vi "Main Application Instance VIs.vi"(8 "Error In":errorcluster, 11 "App In":refnum<vi>) -> (0 "Error Out":errorcluster, 2 "VIs":T1[](array[typedef]), 3 "App Out":refnum<vi>)   [LabVIEW 2017, in "Bookmark Manager.lvlib"]
doc: "According to LabVIEW help: \"LabVIEW also creates a main application instance [MAI], which contains open VIs that are not part of a project and VIs that you did not open from a project.\""
uses:
  Bookmark Manager.lvlib
  Controls/VI Information.ctl
  Controls/Application Information.ctl
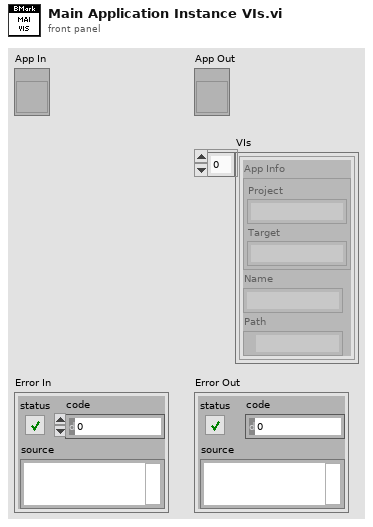
[diagram p1: front panel]
types:
  T1 = typedef "Bookmark Manager.lvlib/VI Information.ctl" = cluster{"App Info":T2, "Name":string, "Path":path}
  T2 = typedef "Bookmark Manager.lvlib/Application Information.ctl" = cluster{"Project":string, "Target":string}
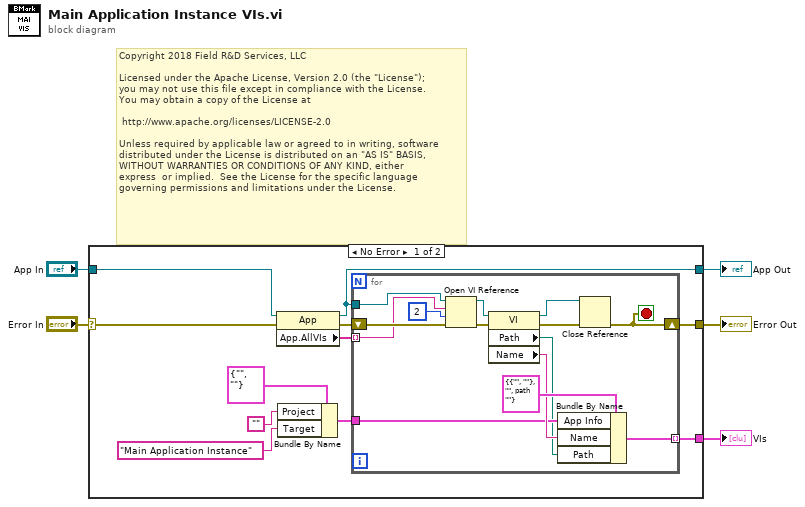
[diagram p0: block diagram]
diagram:
  # "Copyright 2018 Field R&D Services, LLC\n\nLicensed under the Apache License, Version 2.0 (the \"License\");\nyou may not use this file except in compliance with the License.\nYou may obtain a copy of the License at\n\n\thttp://www.apache.org/licenses/LICENSE-2.0\n\nUnless required by applicable law or agreed to in writing, software\ndistributed under the License is distributed on an \"AS IS\" BASIS,\nWITHOUT WARRANTIES OR CONDITIONS OF ANY KIND, either \nexpress  or implied.  See the License for the specific language \ngoverning permissions and limitations under the License."
  n1 = case shown="No Error" "Error In" {
    selector: "Error In" -> [w6 w31]
    tunnel: [w16 w31] -> w5
    tunnel: "App In" -> [w7 w32]
    tunnel: [w13 w32] -> w3
    tunnel: [w12 _] -> w2
    frame No Error {
      n2 = property class="App"(reference=w7, error in=w6) -> (reference out=w13:refnum<vi>, error out=w14:errorcluster, "App.AllVIs"=w15:string[])
      n3 = Bundle By Name(cluster=T2 {"Project"="", "Target"=""} ("App Info"), "Project"="", "Target"="Main Application Instance" ("Project")) -> (w8:T2)
      n4 = for {
        tunnel: w15 -> [w24] mode=indexing
        tunnel: w13 -> [w28]
        tunnel: [w20] -> w12 mode=indexing
        tunnel: w8 -> [w19]
        shift-right: [w18] -> w16
        shift-left: w14 -> [w30]
        stop <- w18 stop-if-true
        n5 = Open VI Reference(application reference (local)=w28, vi path=w24, options=2, error in (no error)=w30) -> (vi reference=w25:refnum<vi>, error out=w29:errorcluster)  [unwired: 2 in]
        n6 = property class="VI"(reference=w25, error in=w29) -> (reference out=w21:refnum<vi>, error out=w26:errorcluster, "Path"=w17:path, "Name"=w22:string)
        n7 = Bundle By Name(cluster=T1 {"App Info"={"Project"="", "Target"=""}, "Name"="", "Path"=path ""} ("VI Info"), "App Info"=w19, "Name"=w22, "Path"=w17) -> (w20:T1)
        n8 = Close Reference(reference=w21, error in (no error)=w26) -> (error out=w18:errorcluster)
      }
    }
    frame Error {
    }
  }
  "Error Out" <- w5
  "VIs" <- w2
  "App Out" <- w3
